vi "InitAction.vi"(6 "InstrumentName":string, 7 "VisaRessIn":refnum<visa-resource-name>, 8 "error in (no error)":errorcluster caption="entrée d'erreur (pas d'erreur)", 9 "FirstClassInst":bool, 10 "Function":string, 11 "GenData In":refnum<class "ThorKDC101.lvclass"> caption="DNL_LabVIEW Object in") -> (0 "error out":errorcluster caption="sortie d'erreur", 3 "GenData Out":refnum<class "ThorKDC101.lvclass"> caption="DNL_LabVIEW Object out")   [LabVIEW 2019, in "ThorKDC101.lvclass"]
uses:
  ThorKDC101.lvclass
  ThorKDC101_Func.ctl
  ThorKDC101.lvclass/ThorKDC101.ctl
panel:
  in  "DefaultDev_Func":T1
  out "VisaRessOut":refnum<visa-resource-name>
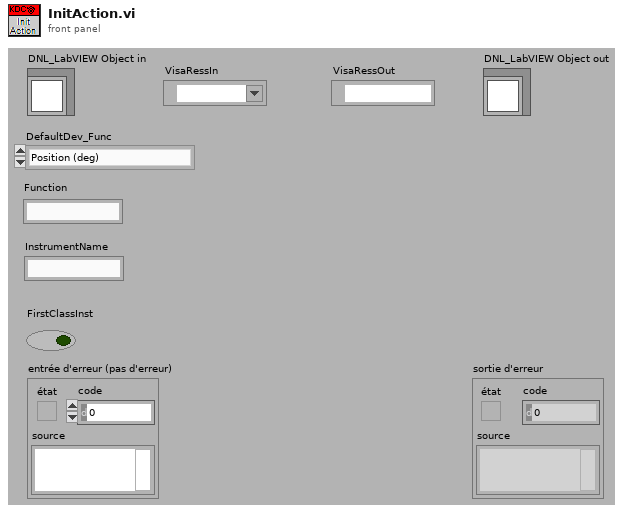
[diagram p1: front panel]
types:
  T1 = typedef "ThorKDC101.lvclass/ThorKDC101_Func.ctl" = enum16{"Position (deg)"}
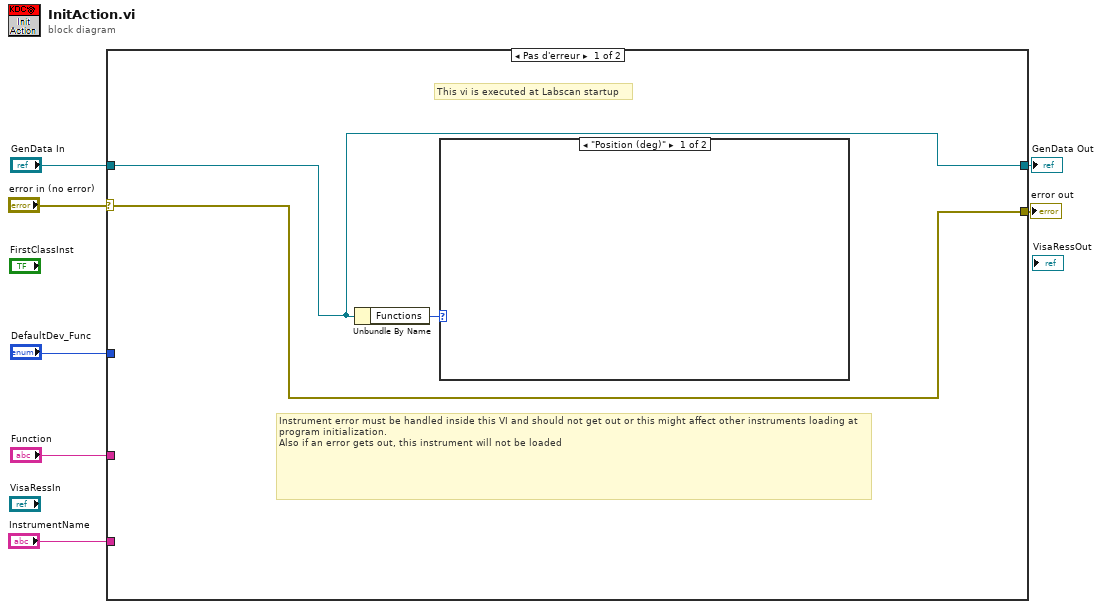
[diagram p0: block diagram]
diagram:
  n1 = case shown="Pas d'erreur" "error in (no error)" {
    selector: "error in (no error)" -> [w8 w12]
    tunnel: [w8 w12] -> w6
    tunnel: "GenData In" -> [w9 w11]
    tunnel: [w9 w11] -> w4
    tunnel: "DefaultDev_Func" -> [_ _]
    tunnel: "Function" -> [_ _]
    tunnel: "InstrumentName" -> [_ _]
    frame No Error {
      # "This vi is executed at Labscan startup"
      # "Instrument error must be handled inside this VI and should not get out or this might affect other instruments loading at program initialization.\nAlso if an error gets out, this instrument will not be loaded"
      n2 = Unbundle By Name(w9) -> ("Functions"=w10:T1)
      n3 = case shown="\"Position (deg)\"" w10 {
        frame "Position (deg)" {
        }
        frame Default {
        }
      }
    }
    frame Error {
    }
  }
  "error out" <- w6
  "GenData Out" <- w4
